vi "Microscope.GetDataValueReference.vi"(11 "Microscope":refnum<class "Microscope.lvclass">) -> (1 "Ref":T1)   [LabVIEW 2013, in "Microscope.lvclass"]
uses:
  Microscope.lvclass
  Typedefs/PrivateData--Ref.ctl
  Typedefs/PrivateData--Cluster.ctl
  Typedefs/PublicEvents--Cluster.ctl
  Typedefs/ValueChanged--EventData--Cluster.ctl
  Typedefs/PublicEvents--Microscope.Initialized.ctl
  Typedefs/ProtectedEvents--Cluster.ctl
  Typedefs/NewValueEvent--Cluster.ctl
  Typedefs/PrivateEvents--Cluster.ctl
  Typedefs/PrivateEvents--Microscope.Initialize.ctl
  Typedefs/PrivateEvents--Microscope.CaptureImageAtPosition.ctl
  XYStage/Typedefs/(real)Coords--Cluster.ctl
  Typedefs/Dependencies--Cluster.ctl
  XYStage/XYStage.lvclass
  Camera/Camera.lvclass
  Typedefs/Configuration--Cluster.ctl
  Microscope.lvclass/Microscope.ctl
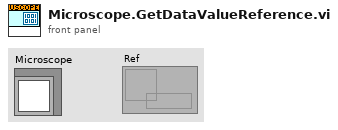
[diagram p1: front panel]
types:
  T1 = typedef "Microscope.lvclass/PrivateData--Ref.ctl" = refnum<data-value>
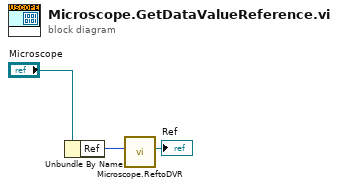
[diagram p0: block diagram]
diagram:
  n1 = Unbundle By Name("Microscope") -> ("Ref"=w2:u32)
  n2 = call "Microscope.ReftoDVR.vi"("Ref"=w2) -> ("Ref"=→"Ref":T1)  [unwired: 10 in]
